vi "config.vi"() -> (3 "info":T1)   [LabVIEW 2015]
uses:
  <vilib>/Utility/config.llb/NI_LVConfig.lvlib
panel:
  in  "error in (no error)":errorcluster
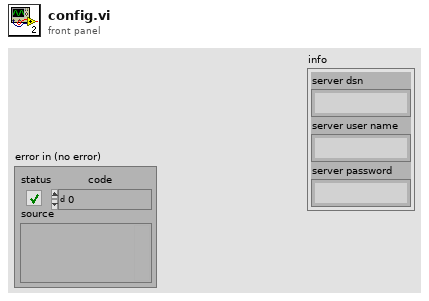
[diagram p1: front panel]
types:
  T1 = cluster{"server dsn":string, "server user name":string, "server password":string}
  T2 = typedef "NI_LVConfig.lvlib/Config Data RefNum.ctl" = refnum<k1>
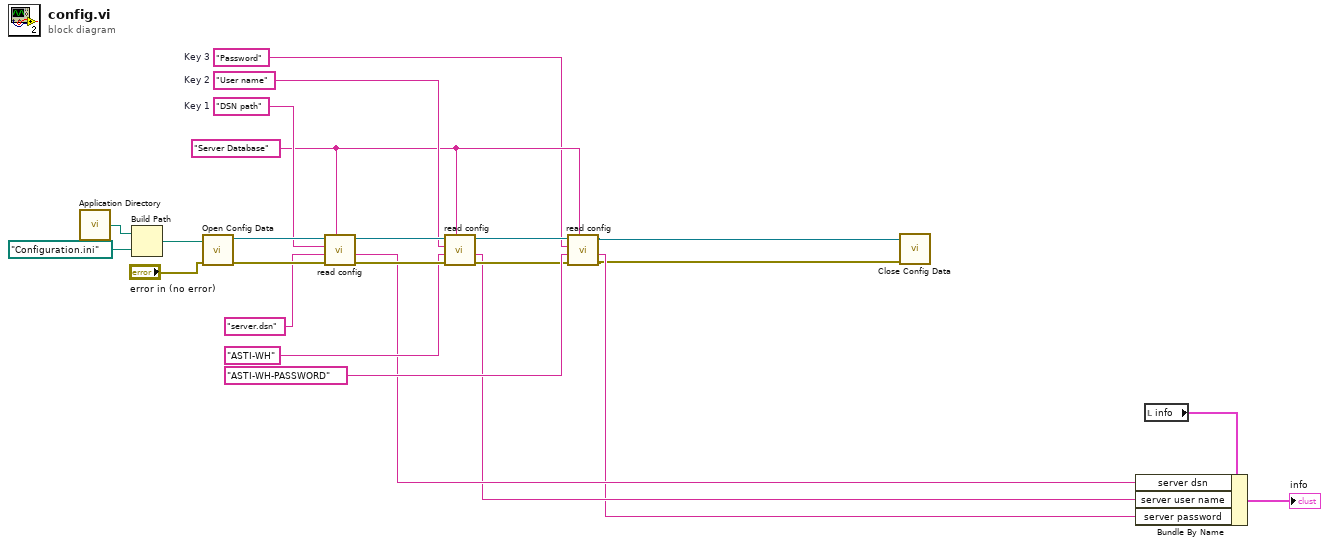
[diagram p0: block diagram]
diagram:
  w9 = "Password"  # Key 3
  w14 = "User name"  # Key 2
  w17 = "DSN path"  # Key 1
  w11 = "Server Database"
  n1 = call <vilib>:"Application Directory.vi"() -> ("Application Directory"=w23:path)
  n2 = Build Path(base path=w23, name or relative path=path "Configuration.ini" ("default name")) -> (appended path=w22:path)
  n3 = call <vilib>:"Open Config Data.vi"("error in (no error)"="error in (no error)", "configuration file path"=w22) -> ("error out"=w19:errorcluster, "refnum"=w20:T2)  [unwired: 1 in, 7 out]
  n4 = call "read config.vi"("Section"=w11, "error in (no error) 2"=w19, "Default value"="server.dsn" ("value"), "Key"=w17, "refnum"=w20) -> ("error out"=w15:errorcluster, "value"=w5:string, "refnum out"=w16:T2)  [unwired: 4 in]
  n5 = call "read config.vi"("Section"=w11, "error in (no error) 2"=w15, "Default value"="ASTI-WH" ("value"), "Key"=w14, "refnum"=w16) -> ("error out"=w8:errorcluster, "value"=w4:string, "refnum out"=w12:T2)  [unwired: 4 in]
  n6 = call "read config.vi"("Section"=w11, "error in (no error) 2"=w8, "Default value"="ASTI-WH-PASSWORD" ("value"), "Key"=w9, "refnum"=w12) -> ("error out"=w1:errorcluster, "value"=w3:string, "refnum out"=w2:T2)  [unwired: 4 in]
  n7 = call <vilib>:"Close Config Data.vi"("error in (no error)"=w1, "refnum"=w2) -> ()  [unwired: 8 in, 2 out]
  n8 = local read "info"() -> (w7:T1)
  n9 = Bundle By Name(cluster=w7, "server dsn"=w5, "server user name"=w4, "server password"=w3) -> (→"info":T1)
